vi "To and From CSV.vi"() -> (0 "error out":errorcluster, 3 "Pass":bool)   [LabVIEW 2015]
uses:
  SystemLink File Module tests.lvlib
  <vilib>/NI/Module Execution Interface/Engine Configuration/engine configuration.lvclass
  <vilib>/NI/Configuration Framework/serializable configuration/NISE_CEF_serializable configuration.lvclass
  module/configuration/SystemLink File configuration.lvclass
  editor node/SystemLink File editor node.lvclass
panel:
  out "Lines":bool
  out "Config":bool
  out "Write Channels":bool
  out "Read Channels":bool
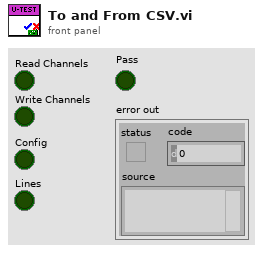
[diagram p1: front panel]
types:
  T1 = typedef "SystemLink File configuration.lvclass/Line.ctl" = cluster{"channel":refnum<class "TBM channel.lvclass">, "Data Tag Type":T2}
  T2 = typedef "SystemLink File configuration.lvclass/Data Tag Type.ctl" = enum16{"Double", "Single", "I32", "I16", "I8", "U64", "U32", "U16", "U8", "Boolean", "String", "Timestamp"}
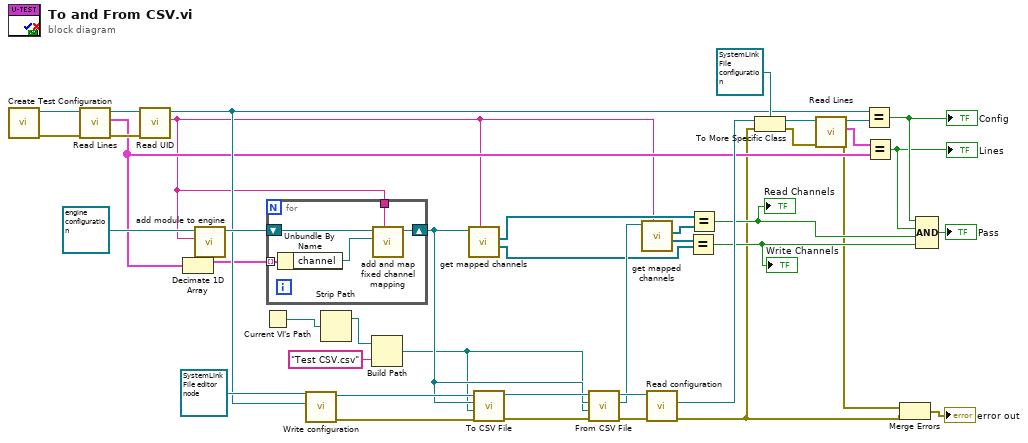
[diagram p0: block diagram]
diagram:
  n1 = call "Create Test Configuration.vi"() -> ("error out"=w20:errorcluster, "Module Configuration"=w21:refnum<class "SystemLink File configuration.lvclass">)  [unwired: 7 in, 3 out]
  n2 = call "Read Lines.vi"("error in (no error)"=w20, "SystemLin Tag Module configuration in"=w21) -> ("error out"=w18:errorcluster, "Lines"=w13:T1[], "SystemLin Tag Module configuration out"=w19:refnum<class "SystemLink File configuration.lvclass">)  [unwired: 7 in]
  n3 = call <vilib>:"Read UID.vi"("error in"=w18, "configuration in"=w19) -> ("instance id"=w5:string, "configuration out"=w15:refnum<class "SystemLink File configuration.lvclass">)  [unwired: 7 in, 1 out]
  n4 = Decimate 1D Array(w13) -> (w4:T1[])  [unwired: 1 out]
  n5 = call-dynamic "add module to engine.vi"("module ID"=w5, "engine configuration in"=refnum<class "engine configuration.lvclass"> refnum ("engine configuration")) -> ("engine configuration out"=w40:refnum<class "engine configuration.lvclass">)  [unwired: 8 in, 1 out]
  n6 = Current VI's Path() -> (path=w24:path)
  n7 = for {
    tunnel: w4 -> [w45] mode=indexing
    shift-right: [w44] -> w26
    shift-left: w40 -> [w43]
    tunnel: w5 -> [w42]
    n8 = Unbundle By Name(w45) -> ("channel"=w46:refnum<class "TBM channel.lvclass">)
    n9 = call <vilib>:"add and map fixed channel mapping.vi"("module instance"=w42, "fixed channel"=w46, "engine configuration in"=w43) -> ("engine configuration out"=w44:refnum<class "engine configuration.lvclass">)  [unwired: 7 in, 1 out]
  }
  n10 = call-dynamic "Write configuration.vi"("configuration"=w15, "SystemLin Tag Module editor node in"=refnum<class "SystemLink File editor node.lvclass"> refnum ("SystemLin Tag Module editor node")) -> ("error out"=w6:errorcluster, "SystemLin Tag Module editor node out"=w38:refnum<class "SystemLink File editor node.lvclass">)  [unwired: 8 in]
  n11 = Strip Path(path=w24) -> (stripped path=w23:path)  [unwired: 1 out]
  n12 = Build Path(base path=w23, name or relative path="Test CSV.csv") -> (appended path=w22:path)
  n13 = call-dynamic "get mapped channels.vi"("owner"=w5, "engine configuration in"=w26) -> ("write channels"=w27:refnum<class "TBM channel.lvclass">[], "read channels"=w29:refnum<class "TBM channel.lvclass">[])  [unwired: 5 in, 3 out]
  n14 = call-dynamic "To CSV File.vi"("error in"=w6, "Path"=w22, "engine configuration"=w26, "SystemLink editor node in"=w38) -> ("error out"=w7:errorcluster, "SystemLink editor node out"=w36:refnum<class "SystemLink File editor node.lvclass">)  [unwired: 6 in]
  n15 = call-dynamic "From CSV File.vi"("error in"=w7, "Path"=w22, "engine in"=w26, "SystemLink editor node in"=w36) -> ("error out"=w17:errorcluster, "engine out"=w31:refnum<class "engine configuration.lvclass">, "SystemLink editor node out"=w37:refnum<class "SystemLink File editor node.lvclass">)  [unwired: 4 in, 1 out]
  n16 = call-dynamic "get mapped channels.vi"("owner"=w5, "engine configuration in"=w31) -> ("write channels"=w28:refnum<class "TBM channel.lvclass">[], "read channels"=w30:refnum<class "TBM channel.lvclass">[])  [unwired: 5 in, 3 out]
  n17 = call-dynamic "Read configuration.vi"("error in"=w17, "SystemLin Tag Module editor node in"=w37) -> ("error out"=w3:errorcluster, "configuration"=w35:refnum<class "NISE_CEF_serializable configuration.lvclass">)  [unwired: 7 in, 1 out]
  n18 = Equal?(x=w28, y=w27) -> (x = y?=w10:bool)
  "Write Channels" <- w10
  n19 = Equal?(x=w29, y=w30) -> (x = y?=w11:bool)
  "Read Channels" <- w11
  n20 = To More Specific Class(target class=refnum<class "SystemLink File configuration.lvclass"> refnum ("SystemLin Tag Module configuration"), reference=w35, error in=w3) -> (specific class reference=w33:refnum<class "SystemLink File configuration.lvclass">, error out=w32:errorcluster)
  n21 = call "Read Lines.vi"("error in (no error)"=w32, "SystemLin Tag Module configuration in"=w33) -> ("error out"=w1:errorcluster, "Lines"=w14:T1[], "SystemLin Tag Module configuration out"=w16:refnum<class "SystemLink File configuration.lvclass">)  [unwired: 7 in]
  n22 = Equal?(x=w15, y=w16) -> (x = y?=w9:bool)
  "Config" <- w9
  n23 = Equal?(x=w14, y=w13) -> (x = y?=w8:bool)
  "Lines" <- w8
  n24 = Merge Errors(w1, w3) -> (→"error out":errorcluster)
  n25 = Compound Arithmetic op=AND(w9, w8, w11, w10) -> (→"Pass":bool)
